vi "Step_valve_fr_server.vi"() -> (0 "Valve Error Info":string, 1 "Output Value":dbl format="%.2f")   [LabVIEW 2014]
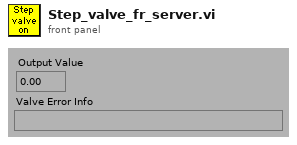
[diagram p1: front panel]
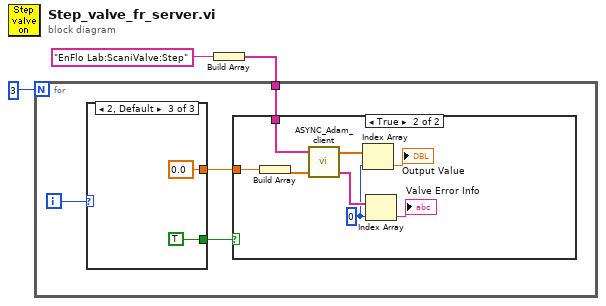
[diagram p0: block diagram]
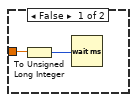
[diagram p2: hidden frame]
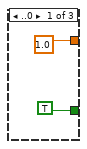
[diagram p3: hidden frame]
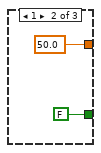
[diagram p4: hidden frame]
diagram:
  n1 = Build Array("EnFlo Lab:ScaniValve:Step") -> (w2:string[])
  n2 = for {
    N: 3 -> [_]
    tunnel: w2 -> [w7]
    i -> [w6]
    n3 = case shown="2, Default" w6 {
      tunnel: [1.0 50.0 ("milliseconds to wait") 0.0 ("milliseconds to wait")] -> w5
      tunnel: [TRUE FALSE TRUE] -> w4
      frame ..0 {
      }
      frame 1 {
      }
      frame 2, Default {
      }
    }
    n4 = case shown="True" w4 {
      tunnel: w7 -> [_ w17]
      tunnel: w5 -> [w9 w16]
      frame False {
        n5 = To Unsigned Long Integer(number=w9) -> (unsigned 32bit integer=w8:u32)
        n6 = Wait (ms)(milliseconds to wait=w8) -> ()  [unwired: 1 out]
      }
      frame True {
        w12 = 0 ("Index")
        n7 = Build Array(w16) -> (w15:dbl[])
        n8 = call "ASYNC_Adam_client.vi"("Values"=w15, "Channel Names"=w17) -> ("Scan Comments"=w13:string[], "Calibrated Units"=w14:dbl[])  [unwired: 1 in]
        n9 = Index Array(array=w14, index=w12) -> (element=→"Output Value":dbl)
        n10 = Index Array(array=w13, index=w12) -> (element=→"Valve Error Info":string)
      }
    }
  }
